vi "通告.vi"(8 "error in (no error)":errorcluster caption="错误输入（无错误）", 10 "采集数据":dbl[](array[numeric]), 11 "数据采集 输入":refnum<class "数据采集.lvclass"> caption="DNL_LabVIEW Object in") -> (0 "error out":errorcluster caption="错误输出", 3 "数据采集 输出":refnum<class "数据采集.lvclass"> caption="DNL_LabVIEW Object out")   [LabVIEW 2013, in "数据采集.lvclass"]
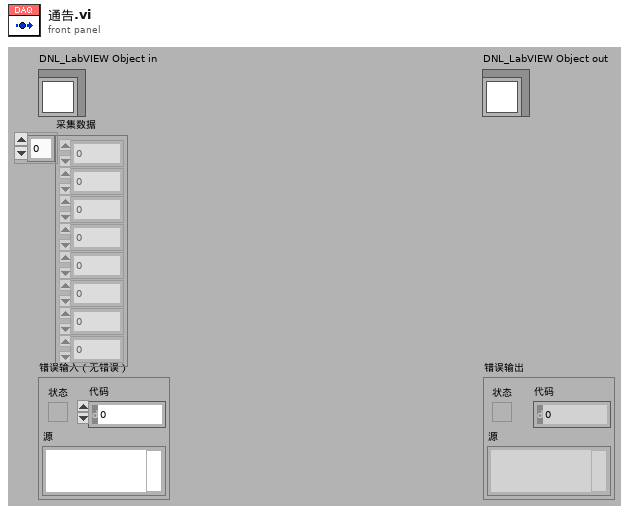
[diagram p1: front panel]
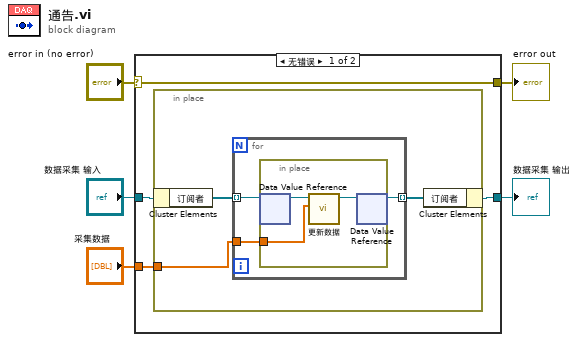
[diagram p0: block diagram]
diagram:
  n1 = case shown="无错误" "error in (no error)" {
    selector: "error in (no error)" -> [w6 w20]
    tunnel: [w6 w20] -> w4
    tunnel: [w7 w19] -> w2
    tunnel: "数据采集 输入" -> [w9 w19]
    tunnel: "采集数据" -> [w8 _]
    frame No Error {
      n2 = in-place {
        in-place-border: w8 -> [w11]
        n3 = in-place-cluster #1(w9) -> ("订阅者"=w12:refnum<data-value>[])
        n4 = for {
          tunnel: [w15] -> w10 mode=indexing
          tunnel: w12 -> [w14] mode=indexing
          tunnel: w11 -> [w13]
          n5 = in-place {
            in-place-border: w13 -> [w16]
            n6 = in-place-dvr #2(w14) -> (w18:refnum<class "订阅者接口.lvclass">)  [unwired: 1 out]
            n7 = call-dynamic "更新数据.vi"("采集数据"=w16, "订阅者接口 输入"=w18) -> ("订阅者接口 输出"=w17:refnum<class "订阅者接口.lvclass">)  [unwired: 8 in, 1 out]
            n8 = in-place-dvr #2(w17) -> (w15:refnum<data-value>)  [unwired: 1 out]
          }
        }
        n9 = in-place-cluster #1("订阅者"=w10) -> (w7:refnum<class "数据采集.lvclass">)
      }
    }
    frame Error {
    }
  }
  "error out" <- w4
  "数据采集 输出" <- w2
